vi "Balls Affect each other.vi"(4 "Numeric":i32, 6 "Cluster":T2, 9 "Array in":T1(array[cluster]), 10 "Boolean":bool, 11 "G":dbl) -> (3 "Array out":T1(array[cluster]))   [LabVIEW 2012]
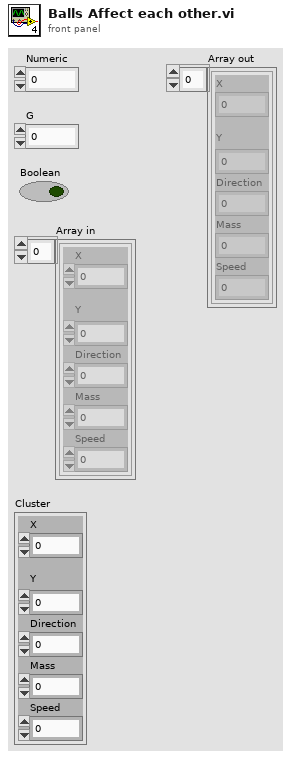
[diagram p1: front panel]
types:
  T1 = cluster{"X":dbl, "\nY":dbl, "Direction":dbl, "Mass":dbl, "Speed":dbl}[]
  T2 = cluster{"X":dbl, "\nY":dbl, "Direction":dbl, "Mass":dbl, "Speed":dbl}
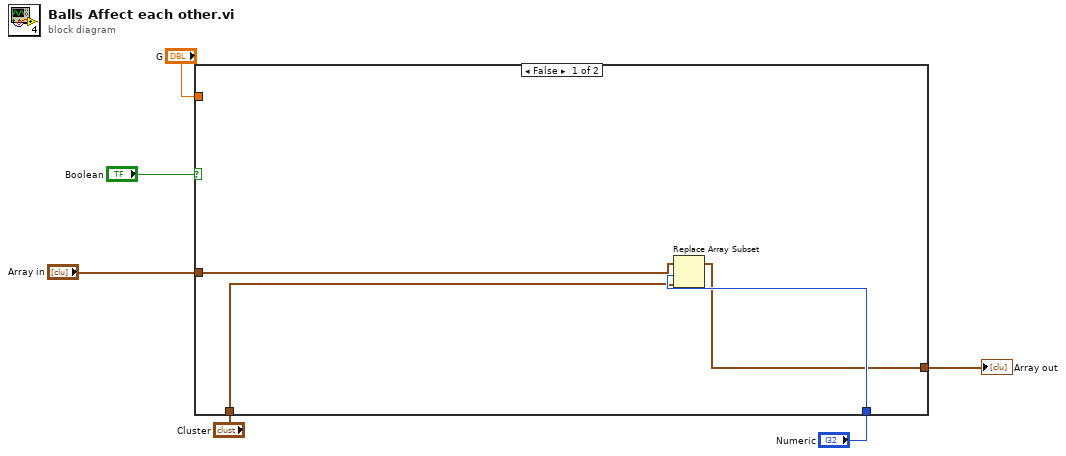
[diagram p0: block diagram]
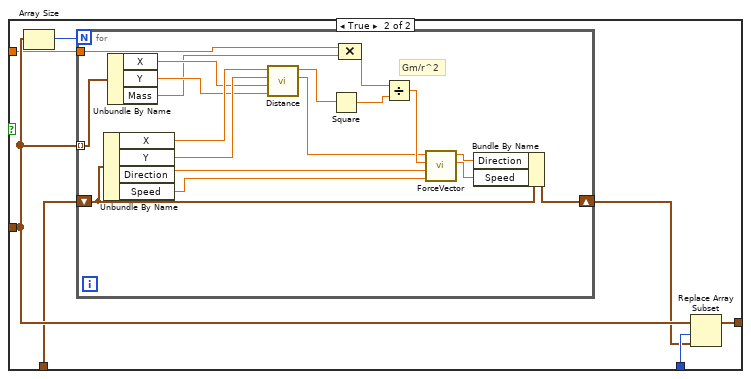
[diagram p2: hidden frame]
diagram:
  n1 = case shown="False" "Boolean" {
    tunnel: [w7 w17] -> w1
    tunnel: "Numeric" -> [w9 w16]
    tunnel: "Array in" -> [w10 w15]
    tunnel: "Cluster" -> [w8 w14]
    tunnel: "G" -> [_ w12]
    frame False {
      n2 = Replace Array Subset(array=w10, new element=w8, index=w9) -> (w7:T1)
    }
    frame True {
      n3 = Array Size(array=w15) -> (size(s)=w11:i32)
      n4 = for {
        N: w11 -> [_]
        tunnel: w15 -> [w32] mode=indexing
        shift-right: [w35] -> w13
        shift-left: w14 -> [w31]
        tunnel: w12 -> [w20]
        # "Gm/r^2"
        n5 = Unbundle By Name(w31) -> ("X"=w28:dbl, "Y"=w27:dbl, "Direction"=w30:dbl, "Speed"=w29:dbl)
        n6 = Unbundle By Name(w32) -> ("X"=w26:dbl, "Y"=w25:dbl, "Mass"=w21:dbl)
        n7 = call "Distance.vi"("Y2"=w25, "X2"=w26, "Y1"=w27, "X1"=w28) -> ("Direction"=w18:dbl, "Distance"=w22:dbl)  [unwired: 6 in]
        n8 = Square(x=w22) -> (x^2=w23:dbl)
        n9 = Compound Arithmetic op=MULTIPLY(w20, w21) -> (w24:dbl)
        n10 = Divide(x=w24, y=w23) -> (x/y=w19:dbl)
        n11 = call "ForceVector.vi"("Vector speed"=w29, "Vector dir"=w30, "Accel"=w19, "Direction"=w18) -> ("Force 2"=w33:dbl, "Direction 2"=w34:dbl)  [unwired: 6 in]
        n12 = Bundle By Name(cluster=w31, "Direction"=w34, "Speed"=w33) -> (w35:T2)
      }
      n13 = Replace Array Subset(array=w15, new element=w13, index=w16) -> (w17:T1)
    }
  }
  "Array out" <- w1
